vi "Read dt.vi"(8 "error in (no error)":errorcluster, 11 "Data1D in":refnum<class "Data1D.lvclass">) -> (0 "error out":errorcluster, 2 "dt":dbl, 3 "Data1D out":refnum<class "Data1D.lvclass">)   [LabVIEW 2014, in "Data1D.lvclass"]
uses:
  Data1D.lvclass
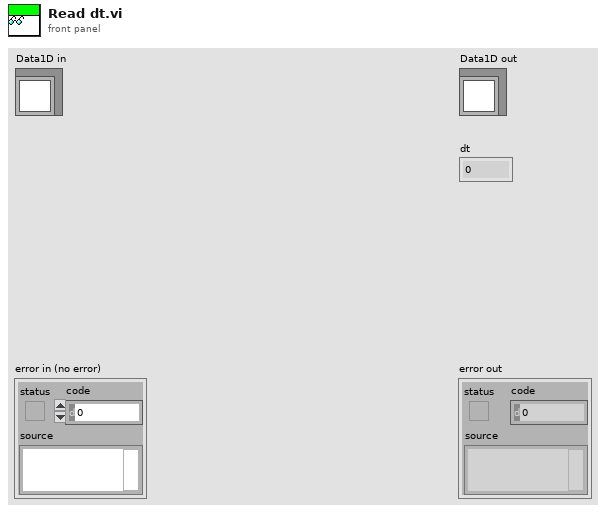
[diagram p1: front panel]
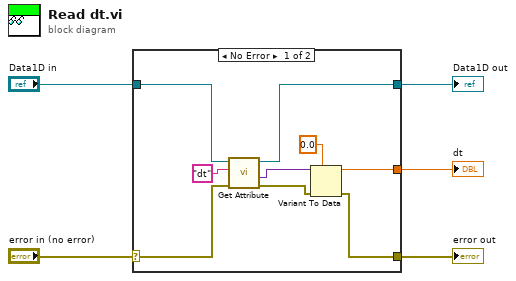
[diagram p0: block diagram]
diagram:
  n1 = case shown="No Error" "error in (no error)" {
    selector: "error in (no error)" -> [w7 w15]
    tunnel: [w12 w15] -> w4
    tunnel: [w10 w16] -> w2
    tunnel: "Data1D in" -> [w11 w16]
    tunnel: [w13 _] -> w1
    frame No Error {
      n2 = call-dynamic "Get Attribute.vi"("error in (no error)"=w7, "Name"="dt", "AbstractData in"=w11) -> ("error out"=w8:errorcluster, "value"=w9:variant, "AbstractData out"=w10:refnum<class "Data1D.lvclass">)  [unwired: 5 in, 1 out]
      n3 = Variant To Data(error in=w8, type=0.0, Variant=w9) -> (data=w13:dbl, error out=w12:errorcluster)
    }
    frame Error {
    }
  }
  "error out" <- w4
  "Data1D out" <- w2
  "dt" <- w1
